vi "SwerveModuleState_Equal.vi"(9 "other SWERVE_DRIVE_MODULE_STATE":T1={"Speed"=0.0, "Angle"={"VALUE"=0.0, "COS"=1.0, "SIN"=0.0}} {"Angle"."SIN" format="%13.4f"; "Angle"."COS" format="%13.4f"; "Angle"."VALUE" format="%13.4f"}, 11 "in SWERVE_DRIVE_MODULE_STATE":T1={"Speed"=0.0, "Angle"={"VALUE"=0.0, "COS"=1.0, "SIN"=0.0}} {"Angle"."SIN" format="%13.4f"; "Angle"."COS" format="%13.4f"; "Angle"."VALUE" format="%13.4f"}) -> (3 "Equal":bool)   [LabVIEW 2019, in "Trajectory_Library.lvlib"]
doc: "Compares two swerve module states. Returns TRUE if they are equal.\n\nParmeters:\n - this Module State\n - other Module State - The other swerve module.\n\nReturns:\n - equal -- boolean -- Returns TRUE if both module states are equal."
uses:
  TypeDef/SWERVE_DRIVE_MODULE_STATE.ctl
  TypeDef/ROTATION2D.ctl
  Trajectory_Library.lvlib
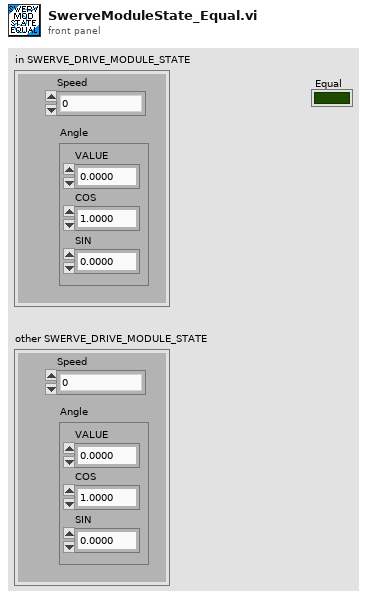
[diagram p1: front panel]
types:
  T1 = typedef "Trajectory_Library.lvlib/SWERVE_DRIVE_MODULE_STATE.ctl" = cluster{"Speed":dbl, "Angle":T2}
  T2 = typedef "Trajectory_Library.lvlib/ROTATION2D.ctl" = cluster{"VALUE":dbl, "COS":dbl, "SIN":dbl}
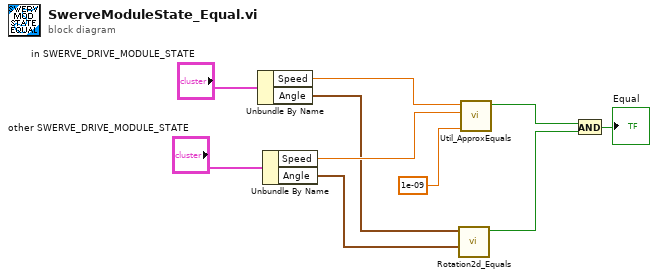
[diagram p0: block diagram]
diagram:
  n1 = Unbundle By Name("in SWERVE_DRIVE_MODULE_STATE") -> ("Speed"=w8:dbl, "Angle"=w3:T2)
  n2 = Unbundle By Name("other SWERVE_DRIVE_MODULE_STATE") -> ("Speed"=w7:dbl, "Angle"=w2:T2)
  n3 = call "Rotation2d_Equals.vi"("other ROTATION"=w2, "in ROTATION"=w3) -> ("Equals"=w1:bool)  [unwired: 9 in]
  n4 = call "Util_ApproxEquals.vi"("Tolerance"=1e-09, "Value 2"=w7, "Value 1"=w8) -> ("ApproxEquals"=w4:bool)  [unwired: 8 in]
  n5 = And(x=w4, y=w1) -> (x .and. y?=→"Equal":bool)
